vi "REACTOR_SECUENCIA_CON_REPETICIONES.vi"(8 "error in (no error)":errorcluster, 9 "SERIAL BRONKHORST":T1, 10 "SERIAL ALICATS":T1) -> (0 "error out":errorcluster, 1 "Secuencia":string[](array[string]), 2 "Sequence":string, 3 "Secuciclos":string[](array[string]), 11 "Path":path=path "C:/Carboquimica 1/Programas")   [LabVIEW 2017]
uses:
  SERIAL ALICATS/__s_TablaAlicats.ctl
panel:
  in  "Up":bool
  out "Repeticiones":bool
  in  "Finalizar":bool
  in  "Borrar":bool
  in  "Grabar Secuencia":bool
  in  "Cargar Secuencia":bool
  out "Fichero":path
  in  "Linea de comando (doble click)":i32(listbox) caption="Válvulas"
  in  "Secuencia":i32(listbox)=-1
  # "Programador de secuencias"
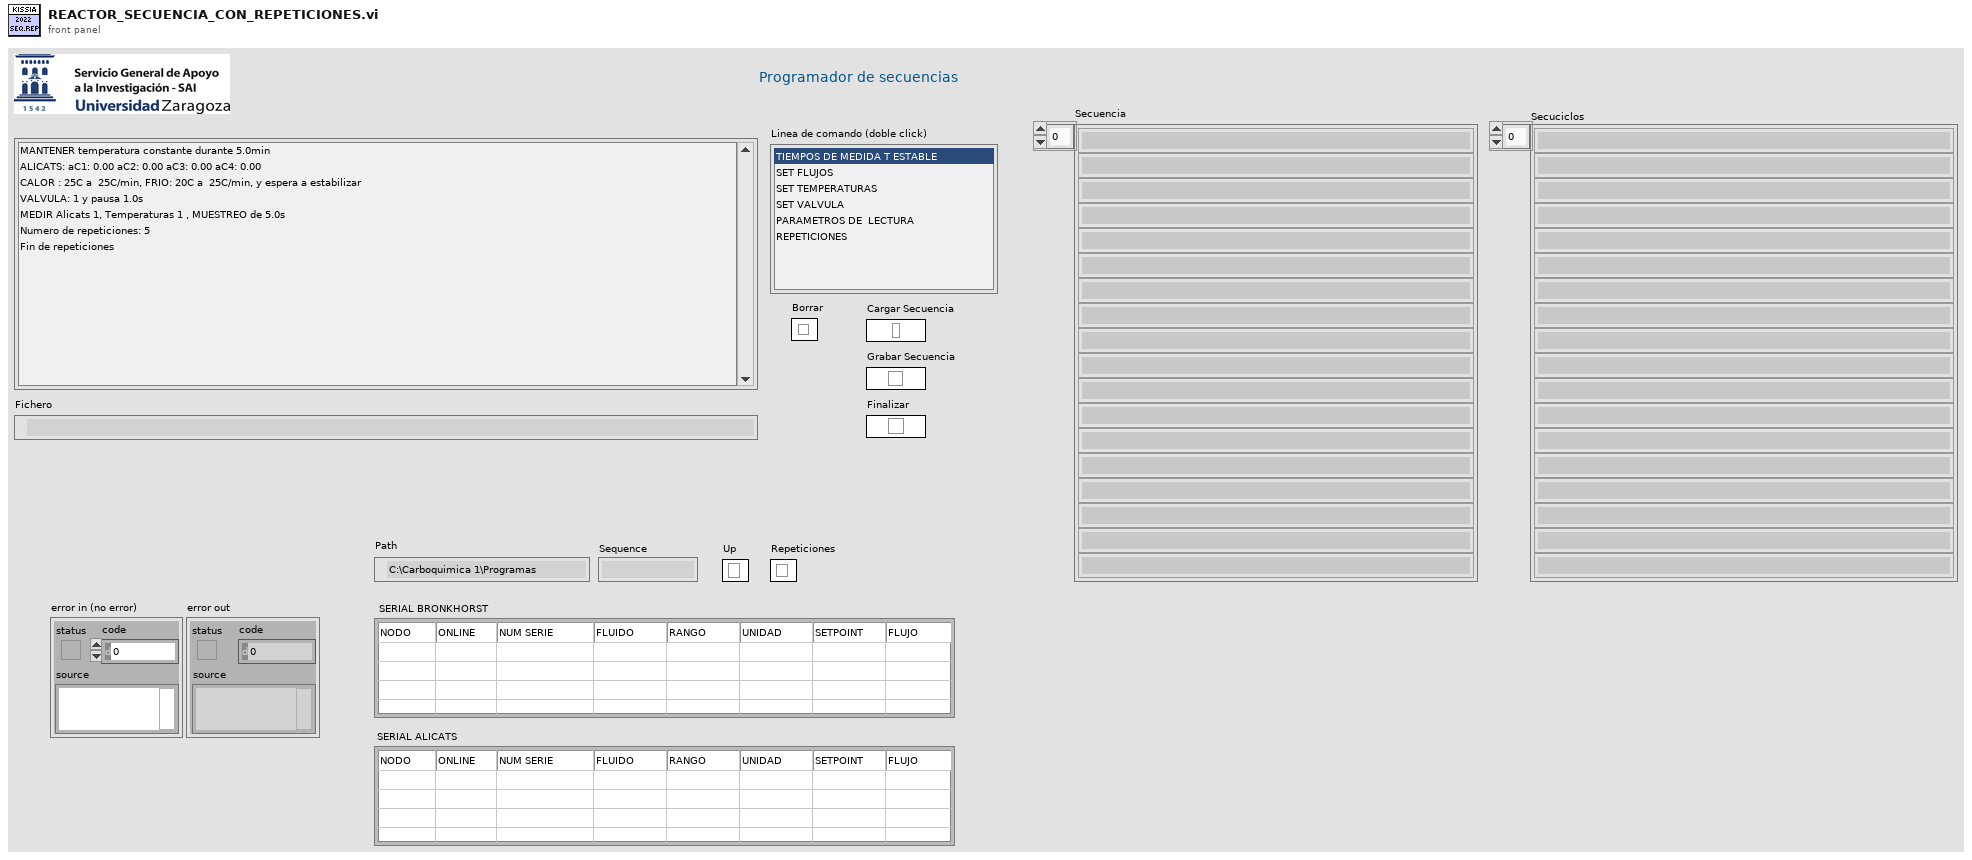
[diagram p1: front panel]
types:
  T1 = typedef "__s_TablaAlicats.ctl" = string[][]
  T2 = enum16{"open", "open or create", "create or replace", "create", "open (read only)"}
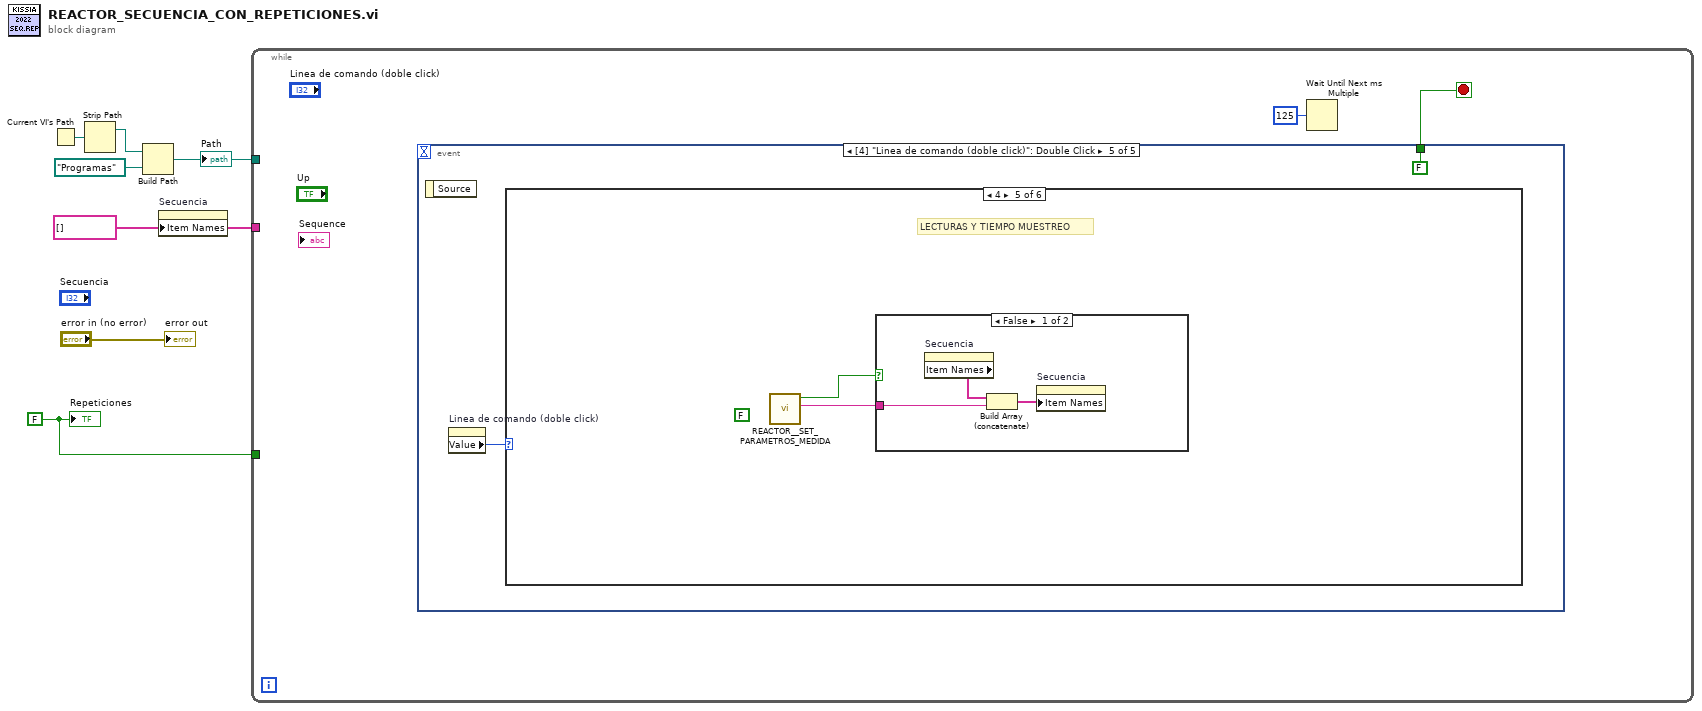
[diagram p0: block diagram]
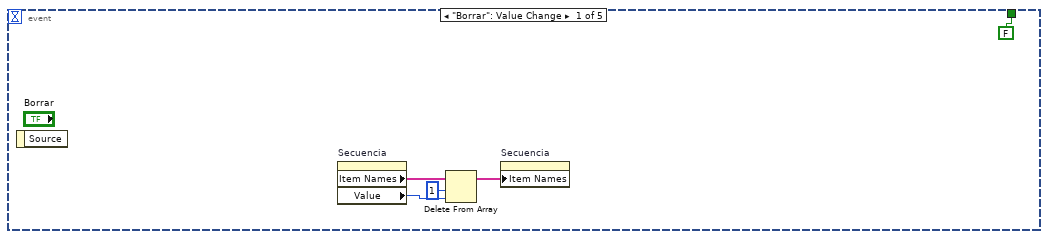
[diagram p2: hidden frame]
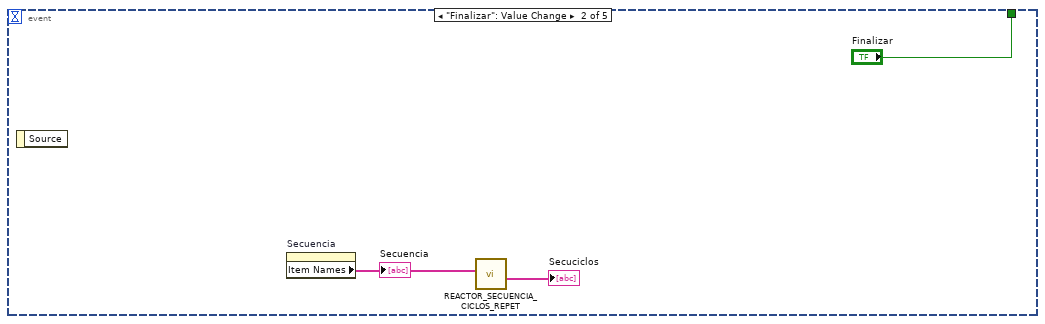
[diagram p3: hidden frame]
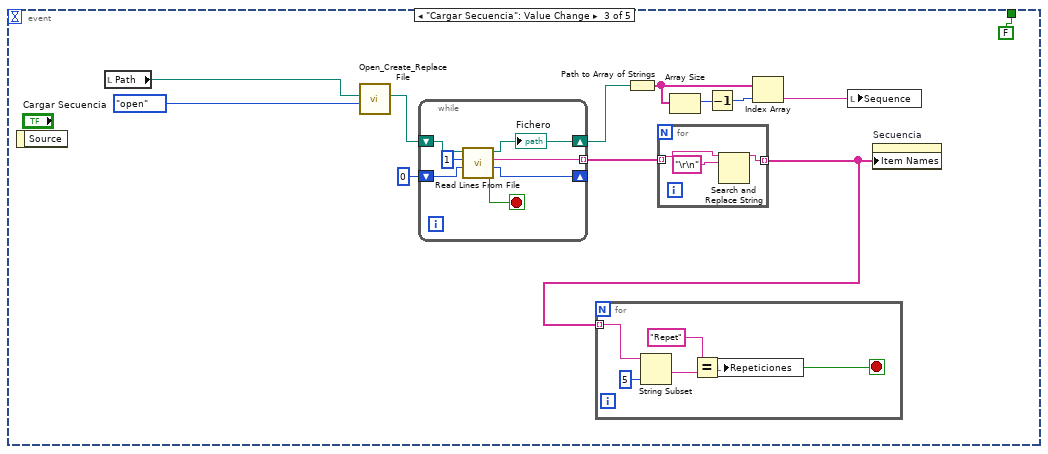
[diagram p4: hidden frame]
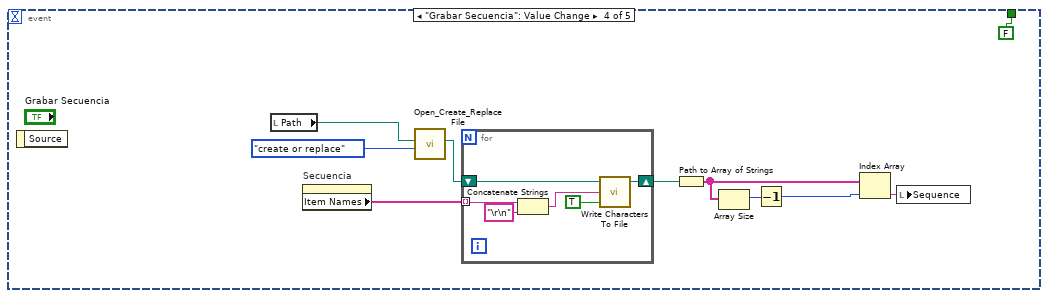
[diagram p5: hidden frame]
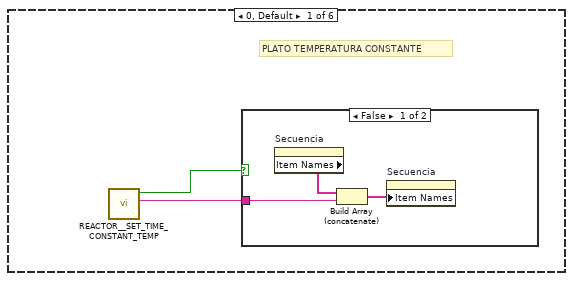
[diagram p6: hidden frame]
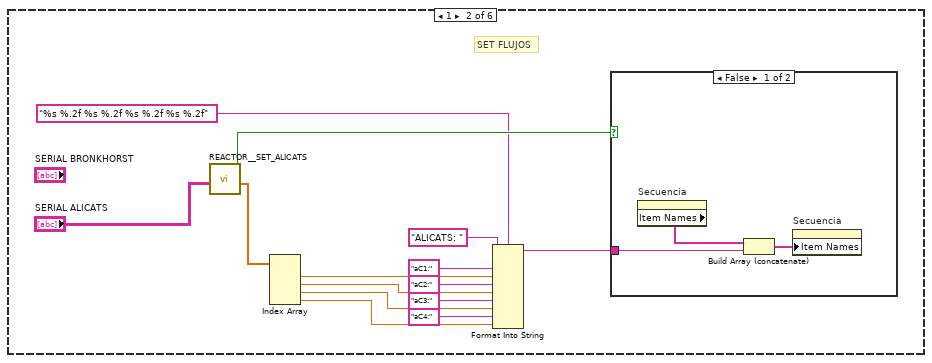
[diagram p8: hidden frame]
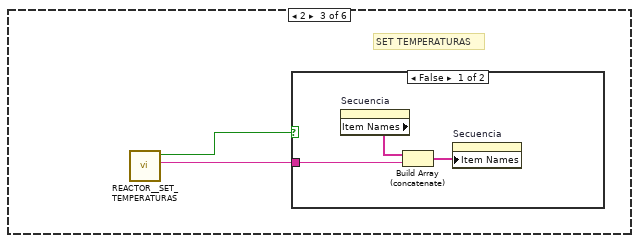
[diagram p10: hidden frame]
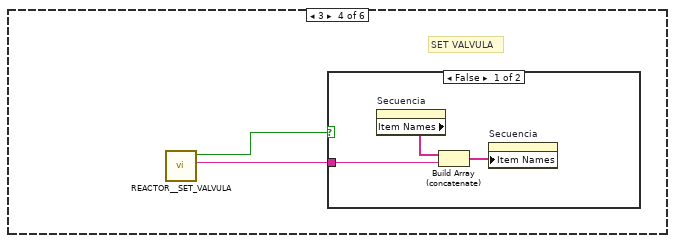
[diagram p12: hidden frame]
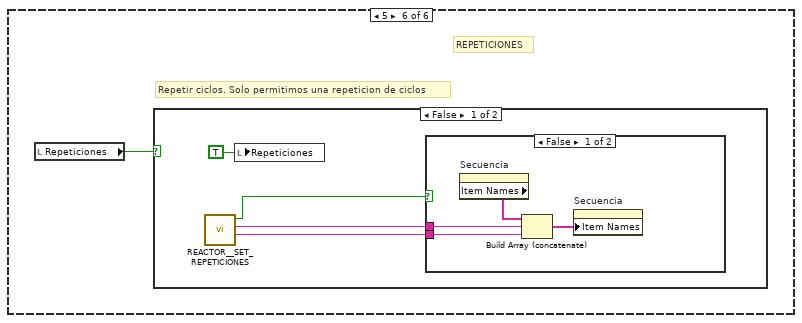
[diagram p15: hidden frame]
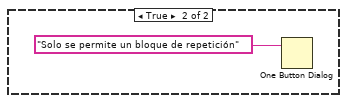
[diagram p17: hidden frame]
diagram:
  w1 = FALSE ("Repeticiones")
  w7 = string[] [] ("Item Names")
  n1 = Current VI's Path() -> (path=w4:path)
  n2 = Strip Path(path=w4) -> (stripped path=w3:path)  [unwired: 1 out]
  n3 = Build Path(base path=w3, name or relative path=path "Programas" ("file path")) -> (appended path=w2:path)
  "Path" <- w2
  n4 = property on="Secuencia" class="LstBox (strict)"("Item Names"=w7) -> ()  [unwired: 2 in, 2 out]
  n5 = while {
    tunnel: w7 -> [_]
    tunnel: w2 -> [_]
    tunnel: w1 -> [_]
    stop <- w8 stop-if-true
    n6 = event shown="[4] \"Linea de comando (doble click)\": Double Click" {
      selector: _ -> [_ _ _ _ _]
      dyn-events: _ -> [_ _ _ _ _]
      timeout: _ -> [_ _ _ _ _]
      tunnel: [FALSE ("Salir") "Finalizar" FALSE ("Salir") FALSE ("Salir") FALSE ("Salir")] -> w8
      event "Borrar": Value Change {
        n7 = event-data() -> ()  [unwired: 1 in, 1 out]
        n8 = property on="Secuencia" class="LstBox (strict)"() -> ("Item Names"=w14:string[], "Value"=w13:i32)  [unwired: 2 in, 2 out]
        n9 = Delete From Array(array=w14, length=1, index=w13) -> (array with subset deleted=w11:string[])  [unwired: 1 out]
        n10 = property on="Secuencia" class="LstBox (strict)"("Item Names"=w11) -> ()  [unwired: 2 in, 2 out]
      }
      event "Finalizar": Value Change {
        n11 = event-data() -> ()  [unwired: 1 in, 1 out]
        n12 = property on="Secuencia" class="LstBox (strict)"() -> ("Item Names"=w16:string[])  [unwired: 2 in, 2 out]
        "Secuencia" <- w16
        n13 = call "REACTOR_SECUENCIA_CICLOS_REPET.vi"("Secuencia"=w16) -> ("Secuciclos"=→"Secuciclos":string[])  [unwired: 9 in, 1 out]
      }
      event "Cargar Secuencia": Value Change {
        n14 = event-data() -> ()  [unwired: 1 in, 1 out]
        n15 = local read "Path"() -> (w20:path)
        n16 = call <vilib>:"Open_Create_Replace File.vi"("function (open:0)"=T2."open", "start path  (Not A Path)"=w20) -> ("new file path"=w27:path)  [unwired: 6 in, 3 out]
        n17 = while {
          shift-right: [w43] -> w21
          shift-left: w27 -> [w44]
          shift-right: [w40] -> _
          shift-left: 0 ("number of lines (all:-1)") -> [w41]
          tunnel: [w38] -> w26 mode=indexing
          stop <- w39 stop-if-true
          n18 = call <vilib>:"Read Lines From File.vi"("file path (dialog if empty)"=w44, "number of lines (all:-1)"=1, "start of read offset (chars.:0)"=w41) -> ("new file path (Not A Path if cancelled)"=w43:path, "line string"=w38:string, "mark after read (chars.)"=w40:i32, "EOF?"=w39:bool)  [unwired: 3 in]
          "Fichero" <- w43
        }
        n19 = Path to Array of Strings(0:w21) -> (2:w25:string[])  [unwired: 1 out]
        n20 = for {
          tunnel: w26 -> [w36] mode=indexing
          tunnel: [w35] -> w18 mode=indexing
          n21 = Search and Replace String(input string=w36, search string="\r\n") -> (result string=w35:string)  [unwired: 6 in, 3 out]
        }
        n22 = for {
          tunnel: w18 -> [w31] mode=indexing
          stop <- w30 stop-if-true
          n23 = String Subset(string=w31, length (rest)=5 ("length (rest)")) -> (substring=w33:string)  [unwired: 1 in]
          n24 = Equal?(x="Repet" ("input 1"), y=w33) -> (x = y?=w30:bool)
          n25 = local write "Repeticiones"(w30) -> ()
        }
        n26 = Array Size(array=w25) -> (size(s)=w24:i32)
        n27 = Decrement(x=w24) -> (x-1=w23:i32)
        n28 = Index Array(array=w25, index=w23) -> (element=w22:string)
        n29 = local write "Sequence"(w22) -> ()
        n30 = property on="Secuencia" class="LstBox (strict)"("Item Names"=w18) -> ()  [unwired: 2 in, 2 out]
      }
      event "Grabar Secuencia": Value Change {
        n31 = event-data() -> ()  [unwired: 1 in, 1 out]
        n32 = local read "Path"() -> (w46:path)
        n33 = property on="Secuencia" class="LstBox (strict)"() -> ("Item Names"=w54:string[])  [unwired: 2 in, 2 out]
        n34 = call <vilib>:"Open_Create_Replace File.vi"("function (open:0)"=T2."create or replace", "start path  (Not A Path)"=w46) -> ("new file path"=w53:path)  [unwired: 6 in, 3 out]
        n35 = for {
          tunnel: w54 -> [w56] mode=indexing
          shift-right: [w59] -> w48
          shift-left: w53 -> [w60]
          n36 = Concatenate Strings(w56, "\r\n") -> (w55:string)
          n37 = call <vilib>:"Write Characters To File.vi"("append to file? (new file:F)"=TRUE, "character string"=w55, "file path (dialog if empty)"=w60) -> ("new file path (Not A Path if cancelled)"=w59:path)  [unwired: 2 in]
        }
        n38 = Path to Array of Strings(0:w48) -> (2:w51:string[])  [unwired: 1 out]
        n39 = Array Size(array=w51) -> (size(s)=w50:i32)
        n40 = Decrement(x=w50) -> (x-1=w49:i32)
        n41 = Index Array(array=w51, index=w49) -> (element=w47:string)
        n42 = local write "Sequence"(w47) -> ()
      }
      event "Linea de comando (doble click)": Double Click {
        n43 = event-data() -> ()  [unwired: 1 in, 1 out]
        n44 = property on="Linea de comando (doble click)" class="LstBox (strict)"() -> ("Value"=w61:i32)  [unwired: 2 in, 2 out]
        n45 = case shown="4" w61 {
          frame 0, Default {
            # "PLATO TEMPERATURA CONSTANTE"
            n46 = call "REACTOR__SET_TIME_CONSTANT_TEMP.vi"() -> ("resulting string 1"=w63:string, "Cancelled?"=w64:bool)  [unwired: 7 in, 1 out]
            n47 = case shown="False" w64 {
              tunnel: w63 -> [w65 _]
              frame False {
                n48 = property on="Secuencia" class="LstBox (strict)"() -> ("Item Names"=w66:string[])  [unwired: 2 in, 2 out]
                n49 = Build Array (concatenate)(w66, w65) -> (w67:string[])
                n50 = property on="Secuencia" class="LstBox (strict)"("Item Names"=w67) -> ()  [unwired: 2 in, 2 out]
              }
              frame True {
              }
            }
          }
          frame 1 {
            # "SET FLUJOS"
            n51 = call "REACTOR__SET_ALICATS.vi"("SERIAL Alicats"="SERIAL ALICATS") -> ("%MFCf"=w74:dbl[], "Cancelled?"=w81:bool)  [unwired: 6 in, 1 out]
            n52 = Index Array(array=w74) -> (element #1=w73:dbl, element #2=w72:dbl, element #3=w71:dbl, element #4=w70:dbl)  [unwired: 4 in]
            n53 = Format Into String(format string="%s %.2f %s %.2f %s %.2f %s %.2f", initial string="ALICATS: " ("message"), "aC1:" ("input 3"), w73, "aC2:" ("input 3"), w72, "aC3:" ("input 5"), w71, "aC4:" ("input 7"), w70) -> (resulting string=w69:string)  [unwired: 1 in, 1 out]
            n54 = case shown="False" w81 {
              tunnel: w69 -> [w83 _]
              frame False {
                n55 = property on="Secuencia" class="LstBox (strict)"() -> ("Item Names"=w82:string[])  [unwired: 2 in, 2 out]
                n56 = Build Array (concatenate)(w82, w83) -> (w84:string[])
                n57 = property on="Secuencia" class="LstBox (strict)"("Item Names"=w84) -> ()  [unwired: 2 in, 2 out]
              }
              frame True {
              }
            }
          }
          frame 2 {
            # "SET TEMPERATURAS"
            n58 = call "REACTOR__SET_TEMPERATURAS.vi"() -> ("resulting string 1"=w85:string, "Cancelled?"=w86:bool)  [unwired: 7 in, 1 out]
            n59 = case shown="False" w86 {
              tunnel: w85 -> [w87 _]
              frame False {
                n60 = property on="Secuencia" class="LstBox (strict)"() -> ("Item Names"=w88:string[])  [unwired: 2 in, 2 out]
                n61 = Build Array (concatenate)(w88, w87) -> (w89:string[])
                n62 = property on="Secuencia" class="LstBox (strict)"("Item Names"=w89) -> ()  [unwired: 2 in, 2 out]
              }
              frame True {
              }
            }
          }
          frame 3 {
            # "SET VALVULA"
            n63 = call "REACTOR__SET_VALVULA.vi"() -> ("resulting string 1"=w90:string, "Cancelled?"=w91:bool)  [unwired: 7 in, 1 out]
            n64 = case shown="False" w91 {
              tunnel: w90 -> [w92 _]
              frame False {
                n65 = property on="Secuencia" class="LstBox (strict)"() -> ("Item Names"=w93:string[])  [unwired: 2 in, 2 out]
                n66 = Build Array (concatenate)(w93, w92) -> (w94:string[])
                n67 = property on="Secuencia" class="LstBox (strict)"("Item Names"=w94) -> ()  [unwired: 2 in, 2 out]
              }
              frame True {
              }
            }
          }
          frame 4 {
            (unwired) FALSE
            # "LECTURAS Y TIEMPO MUESTREO"
            n68 = call "REACTOR__SET_PARAMETROS_MEDIDA.vi"() -> ("resulting string 1"=w95:string, "Cancelled?"=w96:bool)  [unwired: 7 in, 1 out]
            n69 = case shown="False" w96 {
              tunnel: w95 -> [w97 _]
              frame False {
                n70 = property on="Secuencia" class="LstBox (strict)"() -> ("Item Names"=w98:string[])  [unwired: 2 in, 2 out]
                n71 = Build Array (concatenate)(w98, w97) -> (w99:string[])
                n72 = property on="Secuencia" class="LstBox (strict)"("Item Names"=w99) -> ()  [unwired: 2 in, 2 out]
              }
              frame True {
              }
            }
          }
          frame 5 {
            # "REPETICIONES"
            # "Repetir ciclos. Solo permitimos una repeticion de ciclos"
            n73 = local read "Repeticiones"() -> (w100:bool)
            n74 = case shown="False" w100 {
              frame False {
                n75 = call "REACTOR__SET_REPETICIONES.vi"() -> ("resulting string 2"=w102:string, "resulting string 1"=w103:string, "Cancelled?"=w101:bool)  [unwired: 6 in, 1 out]
                n76 = local write "Repeticiones"(TRUE ("Repeticiones")) -> ()
                n77 = case shown="False" w101 {
                  tunnel: w103 -> [w106 _]
                  tunnel: w102 -> [w105 _]
                  frame False {
                    n78 = property on="Secuencia" class="LstBox (strict)"() -> ("Item Names"=w107:string[])  [unwired: 2 in, 2 out]
                    n79 = Build Array (concatenate)(w107, w106, w105) -> (w108:string[])
                    n80 = property on="Secuencia" class="LstBox (strict)"("Item Names"=w108) -> ()  [unwired: 2 in, 2 out]
                  }
                  frame True {
                  }
                }
              }
              frame True {
                n81 = One Button Dialog(message="Solo se permite un bloque de repetición") -> ()  [unwired: 1 in, 1 out]
              }
            }
          }
        }
      }
    }
    n82 = Wait Until Next ms Multiple(millisecond multiple=u32 125) -> ()  [unwired: 1 out]
  }
  "error out" <- "error in (no error)"
  "Repeticiones" <- w1
